vi "file.name_and_type.vi"(10 "File Path":path) -> (1 "File Type":string, 2 "Found":bool, 3 "File Name":string)   [LabVIEW 2020, in "Nominal Client.lvclass"]
doc: "Takes a file path as input and returns the file's MIME type and its name, extracted from the path."
uses:
  Nominal Client.lvclass
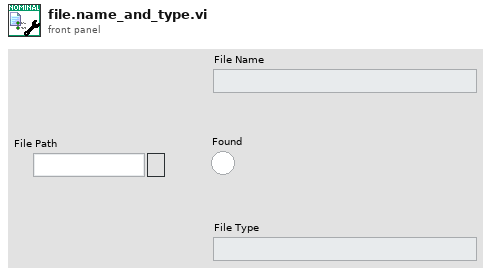
[diagram p1: front panel]
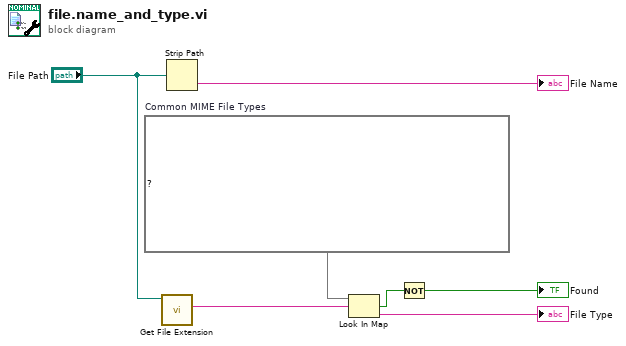
[diagram p0: block diagram]
diagram:
  w5 = map{string, string} {"3gp"="video/3gpp", "7z"="application/x-7z-compressed", "aac"="audio/aac", "amr"="audio/amr", "avi"="video/x-msvideo", "bin"="application/octet-stream", "bmp"="image/bmp", "css"="text/css", "csv"="text/csv", "doc"="application/msword", "docx"="application/vnd.openxmlformats-officedocument.wordprocessingml.document", "flac"="audio/flac", "flv"="video/x-flv", "gif"="image/gif", "gz"="application/gzip", "html"="text/html", "jpg"="image/jpeg", "js"="text/javascript", "json"="application/json", "md"="text/markdown", "midi"="audio/x-midi", "mkv"="video/x-matroska", "mov"="video/quicktime", "mp3"="audio/mpeg", "mp4"="video/mp4", "mpeg"="video/mpeg", "ogg"="audio/ogg", "pdf"="application/pdf", "png"="image/png", "ppt"="application/vnd.ms-powerpoint", "pptx"="application/vnd.openxmlformats-officedocument.presentationml.presentation", "rar"="application/x-rar-compressed", "svg"="image/svg+xml", "swf"="application/x-shockwave-flash", "tar"="application/x-tar", "tiff"="image/tiff", "txt"="text/plain", "wav"="audio/wav", "webm"="video/webm", "wma"="audio/x-ms-wma", "wmv"="video/x-ms-wmv", "xls"="application/vnd.ms-excel", "xlsx"="application/vnd.openxmlformats-officedocument.spreadsheetml.sheet", "xml"="application/xml", "zip"="application/zip"}  # Common MIME File Types
  n1 = call <vilib>:"Get File Extension.vi"("file"="File Path") -> ("lowercase file extension"=w4:string)  [unwired: 6 in, 4 out]
  n2 = Strip Path(path="File Path") -> (name=→"File Name":string)  [unwired: 1 out]
  n3 = Look In Map(map=w5, key=w4) -> (key not found?=w2:bool, value=→"File Type":string)  [unwired: 1 in]
  n4 = Not(x=w2) -> (.not. x?=→"Found":bool)
